vi "CameraVision_Demo_v03.vi"() -> (4 "图像时间戳":u32=16532020 format="%_32g")   [LabVIEW 2015]
uses:
  MVCAMSDK.dll
  <vilib>/Analysis/NI_AALBase.lvlib
  <vilib>/Analysis/NI_AAL_SigProc.lvlib
panel:
  out "泰伯距离数值 3":dbl[](array[numeric])=[15.393849374426454, 15.239052716055017, 15.197063981826837, 15.002070246239633]
  out "Locations 3":dbl[](array[numeric])=[10.438621227921368, 25.832470602347822, 41.07152331840284, 56.268587300229676, 71.27065754646931] caption="上面图像曲线波峰位置"
  out "找到的波谷 2":i32=5
  out "找到的波峰 2":i32=5
  in  "波峰检测器宽度 2":i32=5 min=3
  out "相机每次行进距离  3":dbl=0.1 format="%.2f"
  in  "单次输入步进电机脉冲数  2":i32=20
  out "相机每次行进距离":dbl=0.1 format="%.2f"
  in  "单次输入步进电机脉冲数":i32=20
  out "泰伯距离数值":dbl[](array[numeric])=[15.393849374426454, 15.239052716055017, 15.197063981826837, 15.002070246239633]
  out "Locations":dbl[](array[numeric])=[10.438621227921368, 25.832470602347822, 41.07152331840284, 56.268587300229676, 71.27065754646931] caption="上面图像曲线波峰位置"
  out "找到的波谷":i32=5
  out "找到的波峰":i32=5
  out "信号曲线":cluster{"Locations":dbl[], "Amplitudes":dbl[]}[](graph)=[{"Locations"=array[750 elements], "Amplitudes"=array[749 elements]}, {"Locations"=[104.38621227921368, 258.3247060234782, 410.71523318402836, 562.6858730022967, 712.7065754646931], "Amplitudes"=[11153.698204083417, 10559.387052180104, 10974.865031894917, 10500.852817232146, 11059.763900010517]}, {"Locations"=[26.787398227992274, 182.39455189327623, 333.5517219531509, 488.1851999460032, 636.5270621135614], "Amplitudes"=[3284.809720018355, 2039.4564261182056, 3638.2587716464914, 3082.2730888167225, 4217.856016996603]}]
  in  "波峰检测器宽度":i32=5 min=3
  out "variance 2":dbl caption="方差2" format="%0.2f"
  out "光强图 2":u64[](graph)
  out "variance":dbl caption="方差" format="%0.2f"
  out "相机图像":T1(plugin-control)
  out "光强图":u64[](graph)
  in  "自定义分辨率设置":bool
  in  "ROI分辨率":T2
  in  "预设分辨率设置":bool
  in  "预设分辨率":T3(radio)
  out "帧速":u32
  out "帧间耗时\n单位：（0.1ms）":u32
  in  "相机枚举":T4(ring)
  in  "自动曝光模式":bool=TRUE caption="软触发"
  in  "手动曝光模式":bool caption="软触发"
  in  "曝光时间，单位微秒":dbl=11000.0 format="%#_6f"
  in  "硬触发模式":bool caption="软触发"
  in  "软触发模式":bool caption="软触发"
  in  "连续模式":bool caption="软触发"
  in  "软触发一帧":bool caption="软触发"
  in  "读取自定义数据":bool
  out "从相机中读出的字符串(32字节)":string
  in  "写入自定义数据":bool
  in  "要写入相机的字符串(32字节)":string
  in  "拍照":bool
  in  "相机参数":bool=TRUE
  in  "Stop":bool
  in  "激活预览":bool=TRUE
  out "Image":T1(plugin-control)
  # "相机原生分辨率设置"
  # "写入自定义数据"
  # "触发设置"
  # "曝光设置"
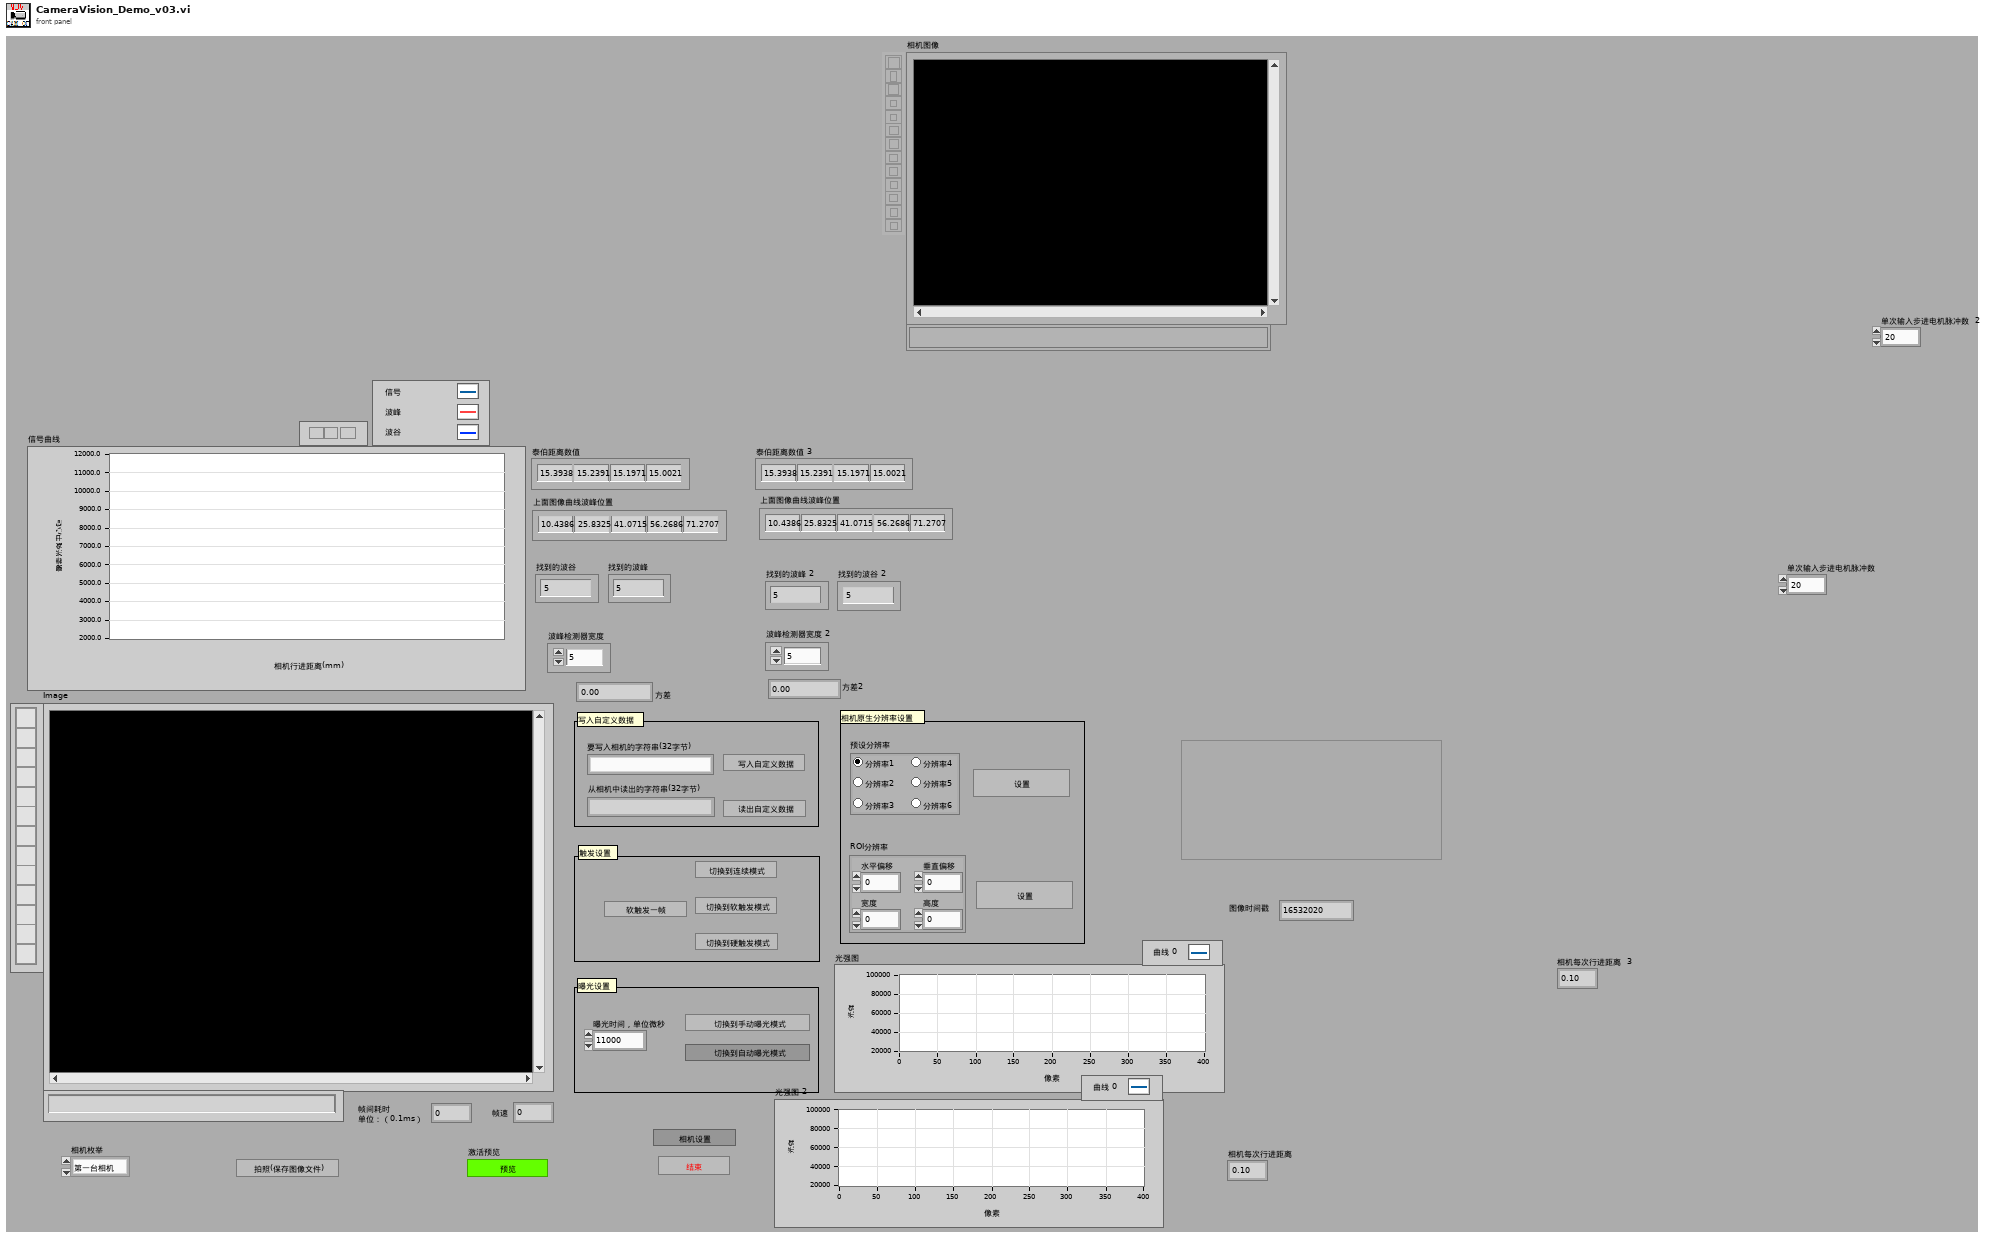
[diagram p1: front panel]
types:
  T1 = typedef "IMAQ Image.ctl" = refnum<image>
  T2 = cluster{"水平偏移":dbl, "垂直偏移":dbl, "宽度":dbl, "高度":dbl}
  T3 = enum32{"分辨率1", "分辨率2", "分辨率3", "分辨率4", "分辨率5", "分辨率6"}
  T4 = enum16{"第一台相机", "第二台相机", "第三台相机", "第四台相机", "第五台相机"}
  T5 = typedef "Image Type" = u32
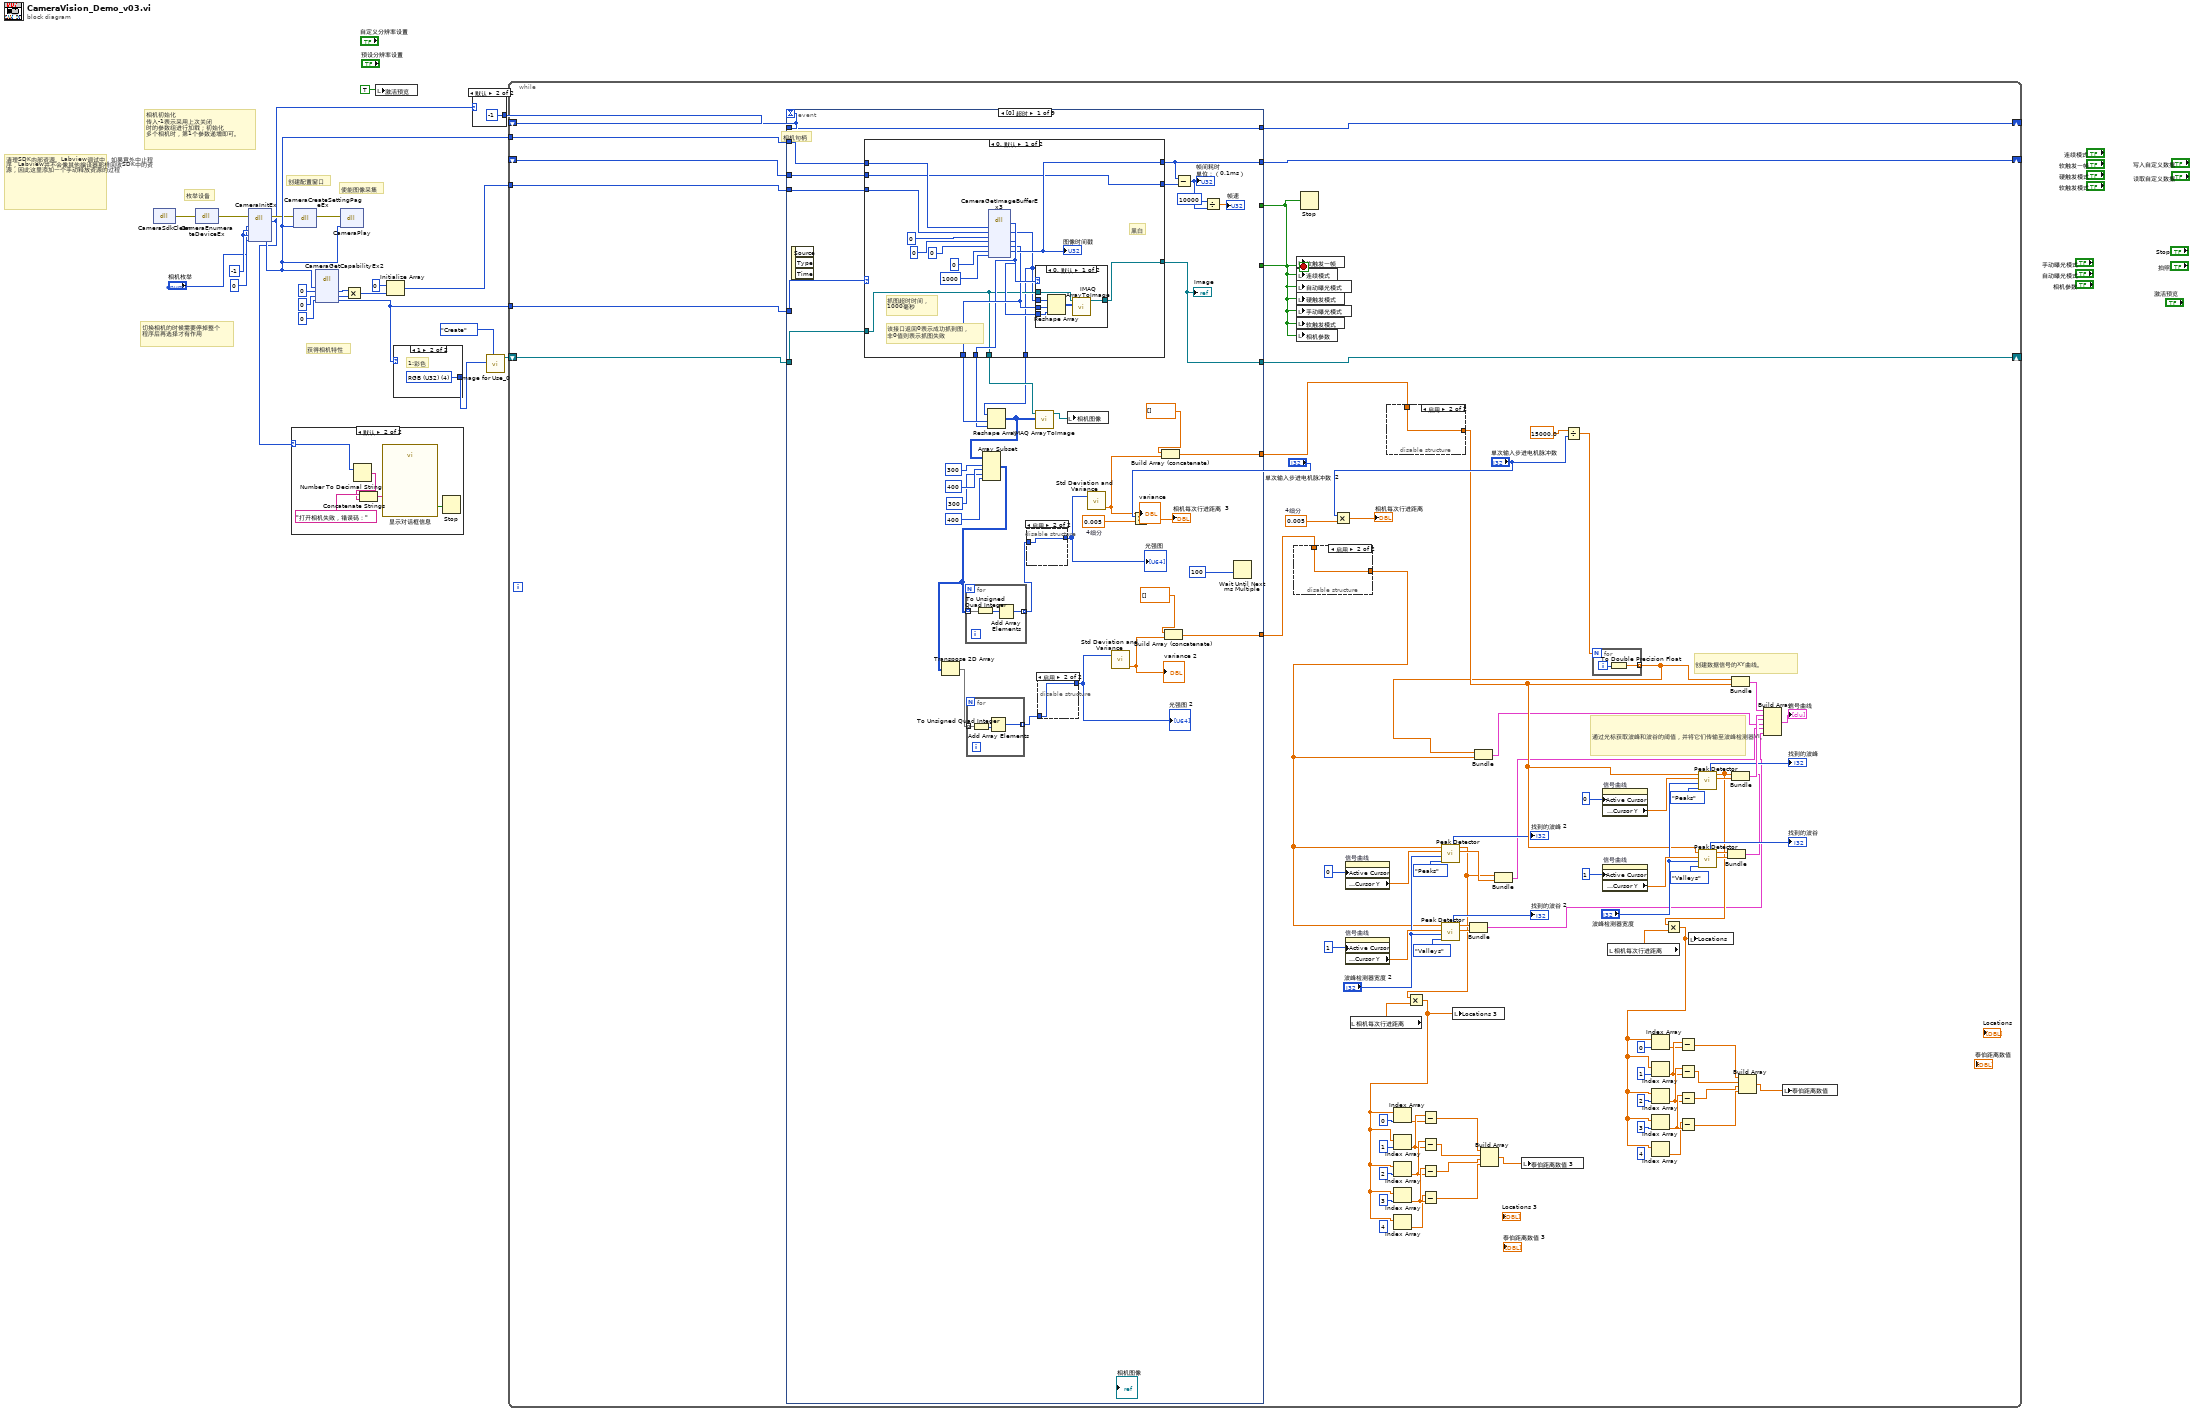
[diagram p0: block diagram]
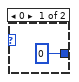
[diagram p2: hidden frame]
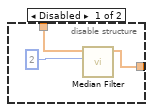
[diagram p4: hidden frame]
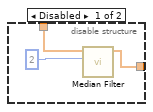
[diagram p5: hidden frame]
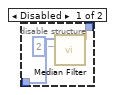
[diagram p6: hidden frame]
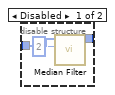
[diagram p7: hidden frame]
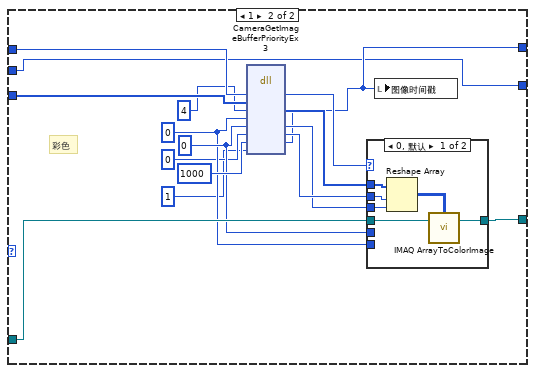
[diagram p9: hidden frame]
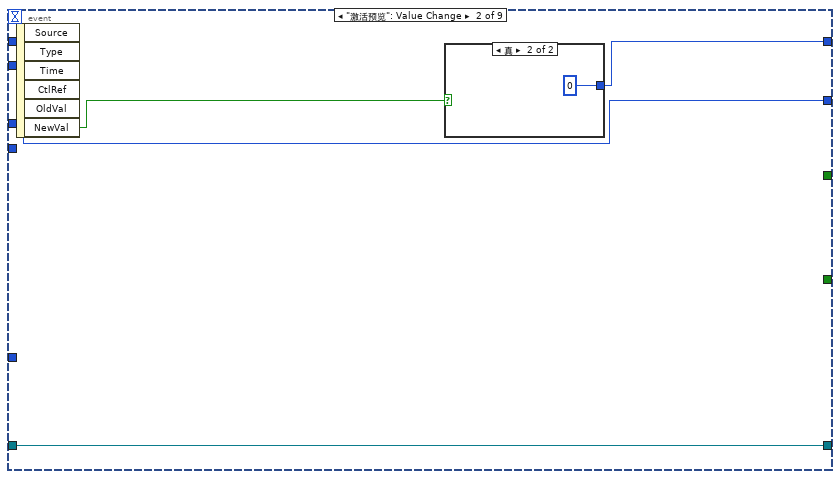
[diagram p11: hidden frame]
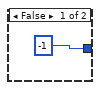
[diagram p12: hidden frame]
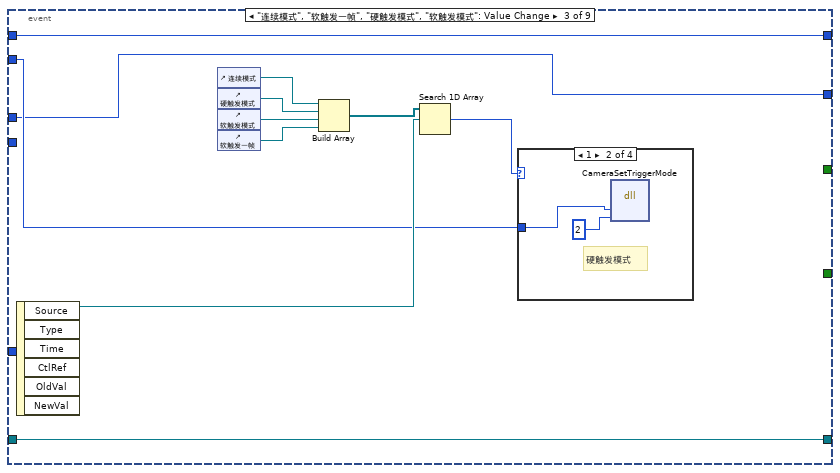
[diagram p13: hidden frame]
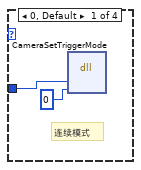
[diagram p14: hidden frame]
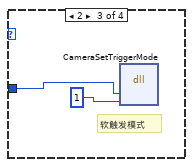
[diagram p15: hidden frame]
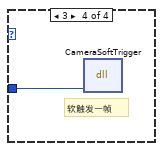
[diagram p16: hidden frame]
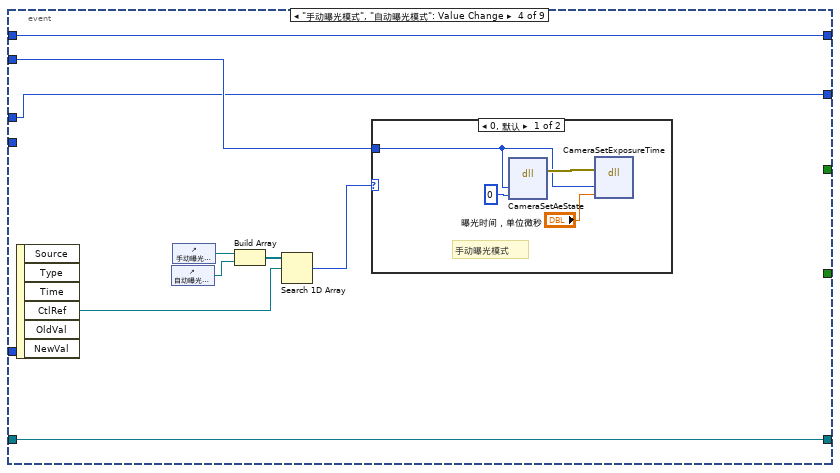
[diagram p17: hidden frame]
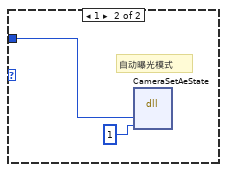
[diagram p18: hidden frame]
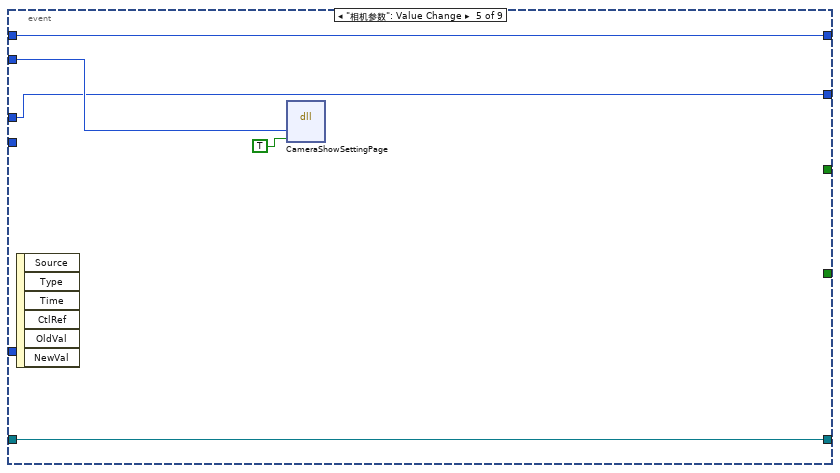
[diagram p19: hidden frame]
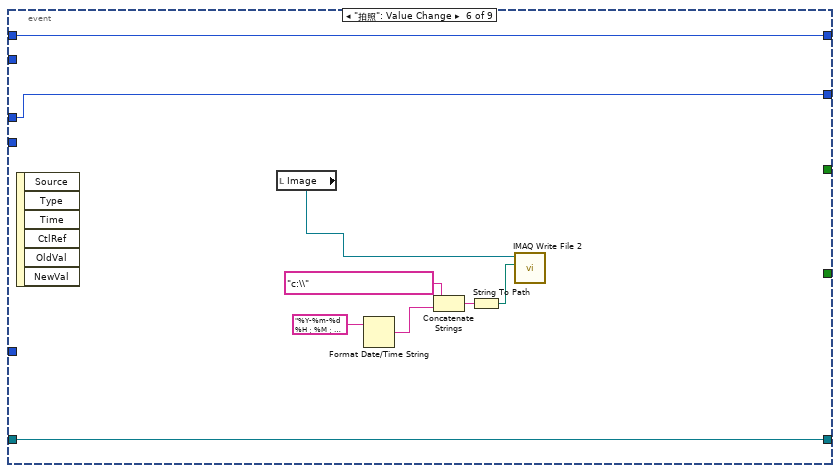
[diagram p20: hidden frame]
diagram:
  w20 = -1
  # "切换相机的时候需要停掉整个\n程序后再选择才有作用"
  # "清理SDK内部资源。Labview调试中，如果意外中止程序，Labview并不会像其他编译器那样回收SDK中的资源，因此这里添加一个手动释放资源的过程"
  # "使能图像采集"
  # "获得相机特性"
  # "创建配置窗口"
  # "相机初始化\n传入-1表示采用上次关闭\n时的参数组进行加载；初始化\n多个相机时，第1个参数递增即可。"
  # "枚举设备"
  n1 = dll-call lib="MVCAMSDK.dll" fn="CameraSdkClean"() -> (error out=w21:errorcluster)  [unwired: 4 in, 1 out]
  n2 = dll-call lib="MVCAMSDK.dll" fn="CameraEnumerateDeviceEx"(error in=w21) -> (error out=w18:errorcluster)  [unwired: 3 in, 1 out]
  n3 = dll-call lib="MVCAMSDK.dll" fn="CameraInitEx"(error in=w18, "相机索引值"="相机枚举", "参数加载方式"=w20, "要加载的参数组索引"=w20, "相机句柄"=0) -> (error out=w7:errorcluster, "返回类型"=w2:i32, "相机句柄"=w9:i32)  [unwired: 5 in, 1 out]
  n4 = case shown="默认" w2 {
    selector: w2 -> [_ w27]
    frame 0 {
    }
    frame Default {
      n5 = Number To Decimal String(number=w27) -> (decimal integer string=w24:string)  [unwired: 1 in]
      n6 = Concatenate Strings("打开相机失败，错误码：" ("字符串"), w24) -> (w26:string)
      n7 = call "显示对话框信息"("Message"=w26) -> ("结束"=w28:bool)  [unwired: 9 in, 1 out]
      n8 = Stop(stop? (T)=w28) -> ()
    }
  }
  n9 = dll-call lib="MVCAMSDK.dll" fn="CameraCreateSettingPageEx"(error in=w7, "相机句柄"=w9) -> (error out=w10:errorcluster)  [unwired: 4 in, 1 out]
  n10 = dll-call lib="MVCAMSDK.dll" fn="CameraGetCapabilityEx2"("相机句柄"=w9, "图像最大宽度"=0, "图像最大高度"=0, "是否是彩色相机(返回0:黑白;1:彩色)"=0) -> ("图像最大宽度"=w12:i32, "图像最大高度"=w11:i32, "是否是彩色相机(返回0:黑白;1:彩色)"=w6:i32)  [unwired: 5 in, 2 out]
  n11 = dll-call lib="MVCAMSDK.dll" fn="CameraPlay"(error in=w10, "相机句柄"=w9) -> ()  [unwired: 4 in, 2 out]
  n12 = Multiply(x=w12, y=w11) -> (x*y=w16:i32)
  n13 = local write "激活预览"(TRUE ("激活预览")) -> ()
  n14 = Initialize Array(0, w16) -> (w8:i32[])
  n15 = case shown="1" w6 {
    tunnel: [_ w29] -> w22
    frame 0, Default {
      # "0:黑白;"
    }
    frame 1 {
      w29 = T5 4 items=["Grayscale (U8)", "Grayscale (I16)", "Grayscale (SGL)", "Complex (CSG)", "RGB (U32)", "HSL (U32)", "RGB (U64)", "Grayscale (U16)"] ("Image Type")
      # "1:彩色"
    }
  }
  n16 = case shown="默认" w2 {
    tunnel: [0 -1] -> w1
    frame 0 {
    }
    frame Default {
    }
  }
  n17 = call "Image for Use_0.vi"("Command"=enum16{"Create", "Use", "Copy in", "Dispose"}."Create", "Image Type"=w22) -> ("Image out"=w5:T1)  [unwired: 8 in, 1 out]
  n18 = while {
    tunnel: w9 -> [w117]
    tunnel: w8 -> [w119]
    tunnel: w6 -> [w120]
    shift-right: [w116] -> _
    shift-left: w1 -> [w115]
    shift-right: [w113] -> _
    shift-left: w5 -> [w118]
    shift-right: [w112] -> _
    shift-left: _ -> [w111]
    stop <- w110 stop-if-true
    (unwired) 4 ("索引")
    w70 = 0.005  # 4细分
    w74 = 0.005  # 4细分
    (unwired) 4 ("索引")
    # "通过光标获取波峰和波谷的阈值，并将它们传输至波峰检测器VI。"
    # "创建数据信号的XY曲线。"
    # "相机句柄"
    n19 = event shown="[0] 超时" {
      selector: _ -> [_ _ _ _ _ _ _ _ _]
      dyn-events: _ -> [_ _ _ _ _ _ _ _ _]
      timeout: w115 -> [_ _ _ _ _ _ _ _ _]
      tunnel: [_ _ _ _ _ _ _ _ TRUE] -> w110
      tunnel: w119 -> [w164 _ _ _ _ _ _ _ _]
      tunnel: w120 -> [w163 _ _ _ _ _ _ _ _]
      tunnel: w117 -> [w165 _ w233 w251 w266 _ w280 w303 w383]
      tunnel: w118 -> [w162 w226 w232 w250 w265 w270 w279 w305 w381]
      tunnel: [w161 w227 w234 w252 w267 w271 w281 w306 w384] -> w116
      tunnel: w115 -> [w161 _ w234 w252 w267 w271 w281 w306 w384]
      tunnel: [_ _ _ _ _ _ _ _ FALSE] -> w114
      tunnel: [w160 w226 w232 w250 w265 w270 w279 w305 w381] -> w113
      tunnel: [w157 w225 w231 w249 w264 w269 w278 w297 w380] -> w112
      tunnel: w111 -> [w159 w225 w231 w249 w264 w269 w278 w297 w380]
      tunnel: [w134 _ _ _ _ _ _ _ _] -> w77
      tunnel: [w131 _ _ _ _ _ _ _ _] -> w67
      event Timeout {
        n20 = event-data() -> ()  [unwired: 1 in, 3 out]
        n21 = case shown="0, 默认" w163 {
          tunnel: w164 -> [w194 w217]
          tunnel: w162 -> [w181 w216]
          tunnel: w165 -> [w186 w215]
          tunnel: [w187 w205] -> w160
          tunnel: [w185 w204] -> w157
          tunnel: w159 -> [w184 w203]
          tunnel: [w184 w203] -> w158
          tunnel: [w183 _] -> w152
          tunnel: [w182 _] -> w151
          tunnel: [w181 _] -> w150
          tunnel: [w180 _] -> w149
          frame 0, Default {
            # "黑白"
            # "该接口返回0表示成功抓到图，\n非0值则表示抓图失败"
            # "抓图超时时间，\n1000毫秒"
            n22 = dll-call lib="MVCAMSDK.dll" fn="CameraGetImageBufferEx3"("相机句柄"=w186, "图像数据缓冲区"=w194, "图像输出格式(0:8位灰度;1:24位彩色;2:32位彩色，3：BGR24彩色 4：BGRA32位彩色)"=0, "图像宽度"=0, "图像高度"=0, "时间戳(单位为100微秒)"=0, "抓图超时时间(毫秒)"=1000) -> ("返回类型"=w189:i32, "图像数据缓冲区"=w180:u8[], "图像宽度"=w182:i32, "图像高度"=w183:i32, "时间戳(单位为100微秒)"=w185:u32)  [unwired: 6 in, 2 out]
            "图像时间戳" <- w185
            n23 = case shown="0, 默认" w189 {
              tunnel: w180 -> [w200 _]
              tunnel: w181 -> [w197 w201]
              tunnel: w183 -> [w199 _]
              tunnel: w182 -> [w198 _]
              tunnel: [w195 w201] -> w187
              frame 0, Default {
                n24 = Reshape Array(w200, w199, w198) -> (w196:u8[][])
                n25 = call "IMAQ ArrayToImage"("Image Pixels (U8)"=w196, "Image"=w197) -> ("Image Out"=w195:T1)  [unwired: 8 in, 1 out]
              }
              frame -12 {
              }
            }
          }
          frame 1 {
            w207 = 0
            w208 = 0
            # "彩色"
            n26 = dll-call lib="MVCAMSDK.dll" fn="CameraGetImageBufferPriorityEx3"("相机句柄"=w215, "图像数据缓冲区"=w217, "图像输出格式(0:8位灰度;1:24位彩色;2:32位彩色)"=4, "图像宽度"=w207, "图像高度"=w208, "时间戳（单位为100微秒）"=0, "抓图超时时间(毫秒)"=1000, "取图优先级(0: 取最旧   1:取最新)"=1) -> ("返回类型"=w209:i32, "图像数据缓冲区"=w212:u32[], "图像宽度"=w210:i32, "图像高度"=w211:i32, "时间戳（单位为100微秒）"=w204:u32)  [unwired: 7 in, 2 out]
            n27 = case shown="0, 默认" w209 {
              tunnel: w212 -> [w222 _]
              tunnel: w216 -> [w221 w224]
              tunnel: w211 -> [w220 _]
              tunnel: w210 -> [w219 _]
              tunnel: w208 -> [_ _]
              tunnel: w207 -> [_ _]
              tunnel: [w218 w224] -> w205
              frame 0, Default {
                n28 = Reshape Array(w222, w220, w219) -> (w223:u32[][])
                n29 = call "IMAQ ArrayToColorImage"("Image Pixels (U32)"=w223, "Image"=w221) -> ("Image Out"=w218:T1)  [unwired: 3 in, 1 out]
              }
              frame -12 {
              }
            }
            n30 = local write "图像时间戳"(w204) -> ()
          }
        }
        "Image" <- w160
        n31 = Reshape Array(w149, w152, w151) -> (w138:u8[][])
        n32 = Array Subset(array=w138, index (row)=300 ("索引"), length (row)=400 ("长度"), index (col)=300 ("长度"), length (col)=400 ("索引")) -> (w137:u8[][])
        n33 = Transpose 2D Array(2D array=w137) -> (transposed array=w145:u8[][])
        n34 = for {
          tunnel: w137 -> [w174] mode=indexing
          tunnel: [w175] -> w147 mode=indexing
          n35 = To Unsigned Quad Integer(1:w174) -> (0:w173:u64[])
          n36 = Add Array Elements(numeric array=w173) -> (sum=w175:u64)
        }
        n37 = for {
          tunnel: w145 -> [w167] mode=indexing
          tunnel: [w168] -> w146 mode=indexing
          n38 = To Unsigned Quad Integer(1:w167) -> (0:w166:u64[])
          n39 = Add Array Elements(numeric array=w166) -> (sum=w168:u64)
        }
        n40 = disable-structure shown="启用" {
          disable-tunnel: w147 -> [w178 w179]
          disable-tunnel: [w176 w179] -> w144
          frame Disabled {
            n41 = call <vilib>:"Median Filter.vi"("left rank"=2, "X"=w178) -> ("Filtered X"=w176:dbl[])  [unwired: 8 in, 1 out]
          }
          frame Enabled {
          }
        }
        "光强图" <- w144
        n42 = call "IMAQ ArrayToImage"("Image Pixels (U8)"=w138, "Image"=w150) -> ("Image Out"=w153:T1)  [unwired: 8 in, 1 out]
        n43 = disable-structure shown="启用" {
          disable-tunnel: w146 -> [w171 w172]
          disable-tunnel: [w169 w172] -> w143
          frame Disabled {
            n44 = call <vilib>:"Median Filter.vi"("left rank"=2, "X"=w171) -> ("Filtered X"=w169:dbl[])  [unwired: 8 in, 1 out]
          }
          frame Enabled {
          }
        }
        "光强图 2" <- w143
        n45 = local write "相机图像"(w153) -> ()
        n46 = call <vilib>:"Std Deviation and Variance.vi"("X"=w144) -> ("variance"=w136:dbl)  [unwired: 1 in, 2 out]
        "variance" <- w136
        n47 = call <vilib>:"Std Deviation and Variance.vi"("X"=w143) -> ("variance"=w132:dbl)  [unwired: 1 in, 2 out]
        "variance 2" <- w132
        n48 = Build Array (concatenate)(dbl[] [], w136) -> (w134:dbl[])
        n49 = Build Array (concatenate)(dbl[] [], w132) -> (w131:dbl[])
        n50 = Subtract(x=w157, y=w158) -> (x-y=w156:u32)
        "帧间耗时\n单位：（0.1ms）" <- w156
        n51 = Divide(x=u32 10000 ("帧间耗时"), y=w156) -> (x/y=→"帧速":dbl)
        n52 = Wait Until Next ms Multiple(millisecond multiple=u32 100 ("毫秒倍数")) -> ()  [unwired: 1 out]
      }
      event "激活预览": Value Change {
        n53 = event-data() -> ("NewVal"=w228:bool)  [unwired: 1 in, 5 out]
        n54 = case shown="真" w228 {
          tunnel: [-1 0] -> w227
          frame False {
          }
          frame True {
          }
        }
      }
      event "连续模式", "软触发一帧", "硬触发模式", "软触发模式": Value Change {
        n55 = event-data() -> ("CtlRef"=w236:refnum<vi>)  [unwired: 1 in, 5 out]
        n56 = control-ref of="连续模式"() -> (w238:refnum<vi>)
        n57 = control-ref of="硬触发模式"() -> (w239:refnum<vi>)
        n58 = control-ref of="软触发模式"() -> (w240:refnum<vi>)
        n59 = control-ref of="软触发一帧"() -> (w241:refnum<vi>)
        n60 = Build Array ("创建数组")(w238, w239, w240, w241) -> (w237:refnum<vi>[])
        n61 = Search 1D Array(1D array=w237, element=w236) -> (index of element=w235:i32)  [unwired: 1 in]
        n62 = case shown="1" w235 {
          tunnel: w233 -> [w242 w244 w246 w248]
          frame 0, Default {
            # "连续模式"
            n63 = dll-call lib="MVCAMSDK.dll" fn="CameraSetTriggerMode"("相机句柄"=w242, "模式"=0) -> ()  [unwired: 6 in, 2 out]
          }
          frame 1 {
            # "硬触发模式"
            n64 = dll-call lib="MVCAMSDK.dll" fn="CameraSetTriggerMode"("相机句柄"=w244, "模式"=2) -> ()  [unwired: 6 in, 2 out]
          }
          frame 2 {
            # "软触发模式"
            n65 = dll-call lib="MVCAMSDK.dll" fn="CameraSetTriggerMode"("相机句柄"=w246, "模式"=1) -> ()  [unwired: 6 in, 2 out]
          }
          frame 3 {
            # "软触发一帧"
            n66 = dll-call lib="MVCAMSDK.dll" fn="CameraSoftTrigger"("相机句柄"=w248) -> ()  [unwired: 5 in, 2 out]
          }
        }
      }
      event "手动曝光模式", "自动曝光模式": Value Change {
        n67 = event-data() -> ("CtlRef"=w255:refnum<vi>)  [unwired: 1 in, 5 out]
        n68 = control-ref of="自动曝光模式"() -> (w253:refnum<vi>)
        n69 = control-ref of="手动曝光模式"() -> (w256:refnum<vi>)
        n70 = Build Array ("创建数组")(w256, w253) -> (w257:refnum<vi>[])
        n71 = Search 1D Array(1D array=w257, element=w255) -> (index of element=w254:i32)  [unwired: 1 in]
        n72 = case shown="0, 默认" w254 {
          tunnel: w251 -> [w258 w262]
          frame 0, Default {
            # "手动曝光模式"
            n73 = dll-call lib="MVCAMSDK.dll" fn="CameraSetAeState"("相机句柄"=w258, "曝光模式(0手动，1自动)"=0) -> (error out=w261:errorcluster)  [unwired: 6 in, 1 out]
            n74 = dll-call lib="MVCAMSDK.dll" fn="CameraSetExposureTime"(error in=w261, "相机句柄"=w258, "曝光时间，单位微秒"="曝光时间，单位微秒") -> ()  [unwired: 5 in, 2 out]
          }
          frame 1 {
            # "自动曝光模式"
            n75 = dll-call lib="MVCAMSDK.dll" fn="CameraSetAeState"("相机句柄"=w262, "曝光模式(0手动，1自动)"=1) -> ()  [unwired: 6 in, 2 out]
          }
        }
      }
      event "相机参数": Value Change {
        n76 = event-data() -> ()  [unwired: 1 in, 6 out]
        n77 = dll-call lib="MVCAMSDK.dll" fn="CameraShowSettingPage"("相机句柄"=w266, "状态"=TRUE) -> ()  [unwired: 6 in, 2 out]
      }
      event "拍照": Value Change {
        n78 = event-data() -> ()  [unwired: 1 in, 6 out]
        n79 = local read "Image"() -> (w272:T1)
        n80 = Format Date/Time String(time format string (%c)="%Y-%m-%d %H：%M：%S.bmp ") -> (date/time string=w276:string)  [unwired: 2 in]
        n81 = Concatenate Strings("c:\\", w276) -> (w273:string)
        n82 = String To Path(string=w273) -> (path=w275:path)
        n83 = call-poly "IMAQ Write File 2"("File Path"=w275, "Image"=w272) -> ()  [unwired: 8 in, 2 out]
      }
      event "写入自定义数据", "读取自定义数据": Value Change {
        n84 = event-data() -> ("CtlRef"=w283:refnum<vi>)  [unwired: 1 in, 5 out]
        n85 = control-ref of="读取自定义数据"() -> (w285:refnum<vi>)
        n86 = control-ref of="写入自定义数据"() -> (w284:refnum<vi>)
        n87 = Build Array ("创建数组")(w285, w284) -> (w286:refnum<vi>[])
        n88 = Search 1D Array(1D array=w286, element=w283) -> (index of element=w282:i32)  [unwired: 1 in]
        n89 = case shown="0, 默认" w282 {
          tunnel: w280 -> [w287 w294]
          frame 0, Default {
            n90 = Initialize Array(0, 32) -> (w291:i32[])
            n91 = dll-call lib="MVCAMSDK.dll" fn="CameraReadSN"("相机句柄"=w287, "序列号"=w291, "序列号级别，[0,1,2],0级为只读，1,2级可写"=1) -> ("序列号"=w289:u8[])  [unwired: 6 in, 2 out]
            n92 = Byte Array To String(unsigned byte array=w289) -> (string=→"从相机中读出的字符串(32字节)":string)
          }
          frame 1 {
            n93 = dll-call lib="MVCAMSDK.dll" fn="CameraWriteSN"("相机句柄"=w294, "序列号(固定为32个字节)"="要写入相机的字符串(32字节)", "序列号级别，[0,1,2]对应3级序列号，其中0级为只读，1,2级可写"=1) -> ()  [unwired: 7 in, 2 out]
          }
        }
      }
      event "预设分辨率设置", "自定义分辨率设置": Value Change {
        n94 = event-data() -> ("CtlRef"=w299:refnum<vi>)  [unwired: 1 in, 5 out]
        n95 = control-ref of="预设分辨率设置"() -> (w301:refnum<vi>)
        n96 = control-ref of="自定义分辨率设置"() -> (w300:refnum<vi>)
        n97 = Build Array ("创建数组")(w301, w300) -> (w302:refnum<vi>[])
        n98 = Search 1D Array(1D array=w302, element=w299) -> (index of element=w298:i32)  [unwired: 1 in]
        n99 = case shown="1" w298 {
          tunnel: "预设分辨率" -> [w308 _]
          tunnel: w303 -> [w307 w369]
          frame 0, Default {
            n100 = case shown="\"分辨率2\"" w308 {
              tunnel: w307 -> [w309 w328 w329 w339 w349 w359]
              frame "分辨率1", Default {
                n101 = dll-call lib="MVCAMSDK.dll" fn="CameraSetImageResolutionEx"("相机句柄"=w309, "预设分辨率索引"=0, "Mode"=0, "ModeSize"=u32 0, "x"=0, "y"=u32 0 ("ModeSize"), "width"=0, "height"=0, "ZoomWidth"=0, "ZoomHeight"=0) -> ()  [unwired: 14 in, 2 out]
              }
              frame "分辨率2" {
                n102 = dll-call lib="MVCAMSDK.dll" fn="CameraSetImageResolutionEx"("相机句柄"=w328, "预设分辨率索引"=1, "Mode"=0, "ModeSize"=u32 0, "x"=0, "y"=u32 0 ("ModeSize"), "width"=0, "height"=0, "ZoomWidth"=0, "ZoomHeight"=0) -> ()  [unwired: 14 in, 2 out]
              }
              frame "分辨率3" {
                n103 = dll-call lib="MVCAMSDK.dll" fn="CameraSetImageResolutionEx"("相机句柄"=w329, "预设分辨率索引"=2, "Mode"=0, "ModeSize"=u32 0, "x"=0, "y"=u32 0 ("ModeSize"), "width"=0, "height"=0, "ZoomWidth"=0, "ZoomHeight"=0) -> ()  [unwired: 14 in, 2 out]
              }
              frame "分辨率4" {
                n104 = dll-call lib="MVCAMSDK.dll" fn="CameraSetImageResolutionEx"("相机句柄"=w339, "预设分辨率索引"=3, "Mode"=0, "ModeSize"=u32 0, "x"=0, "y"=u32 0 ("ModeSize"), "width"=0, "height"=0, "ZoomWidth"=0, "ZoomHeight"=0) -> ()  [unwired: 14 in, 2 out]
              }
              frame "分辨率5" {
                n105 = dll-call lib="MVCAMSDK.dll" fn="CameraSetImageResolutionEx"("相机句柄"=w349, "预设分辨率索引"=4, "Mode"=0, "ModeSize"=u32 0, "x"=0, "y"=u32 0 ("ModeSize"), "width"=0, "height"=0, "ZoomWidth"=0, "ZoomHeight"=0) -> ()  [unwired: 14 in, 2 out]
              }
              frame "分辨率6" {
                n106 = dll-call lib="MVCAMSDK.dll" fn="CameraSetImageResolutionEx"("相机句柄"=w359, "预设分辨率索引"=5, "Mode"=0, "ModeSize"=u32 0, "x"=0, "y"=u32 0 ("ModeSize"), "width"=0, "height"=0, "ZoomWidth"=0, "ZoomHeight"=0) -> ()  [unwired: 14 in, 2 out]
              }
            }
          }
          frame 1 {
            n107 = Unbundle("ROI分辨率") -> ("水平偏移"=w371:dbl, "垂直偏移"=w372:dbl, "宽度"=w373:dbl, "高度"=w374:dbl)
            n108 = dll-call lib="MVCAMSDK.dll" fn="CameraSetImageResolutionEx"("相机句柄"=w369, "预设分辨率索引"=255, "Mode"=0, "ModeSize"=u32 0, "x"=w371, "y"=w372, "width"=w373, "height"=w374, "ZoomWidth"=0, "ZoomHeight"=u32 0 ("ModeSize")) -> ()  [unwired: 14 in, 2 out]
          }
        }
      }
      event "Stop": Value Change {
        # "反初始化相机"
        n109 = event-data() -> ()  [unwired: 1 in, 6 out]
        n110 = dll-call lib="MVCAMSDK.dll" fn="CameraUnInit"("相机句柄"=w383) -> ()  [unwired: 5 in, 2 out]
      }
    }
    n111 = Multiply(x="单次输入步进电机脉冲数  2", y=w70) -> (x*y=→"相机每次行进距离  3":dbl)
    n112 = disable-structure shown="启用" {
      disable-tunnel: w67 -> [w122 w124]
      disable-tunnel: [w121 w124] -> w36
      frame Disabled {
        n113 = call <vilib>:"Median Filter.vi"("left rank"=2, "X"=w122) -> ("Filtered X"=w121:dbl[])  [unwired: 8 in, 1 out]
      }
      frame Enabled {
      }
    }
    n114 = local write "软触发一帧"(w114) -> ()
    n115 = local write "连续模式"(w114) -> ()
    n116 = local write "自动曝光模式"(w114) -> ()
    n117 = local write "硬触发模式"(w114) -> ()
    n118 = local write "手动曝光模式"(w114) -> ()
    n119 = local write "软触发模式"(w114) -> ()
    n120 = local write "相机参数"(w114) -> ()
    n121 = Stop(stop? (T)=w110) -> ()
    n122 = Multiply(x="单次输入步进电机脉冲数", y=w74) -> (x*y=→"相机每次行进距离":dbl)
    n123 = property on="信号曲线" class="XYGraph (严格)"("Active Cursor"=u32 0) -> ("Cursor.Cursor Position:Cursor Y"=w60:dbl)  [unwired: 2 in, 2 out]
    n124 = property on="信号曲线" class="XYGraph (严格)"("Active Cursor"=u32 1) -> ("Cursor.Cursor Position:Cursor Y"=w59:dbl)  [unwired: 2 in, 2 out]
    n125 = local read "相机每次行进距离"() -> (w53:dbl)
    n126 = disable-structure shown="启用" {
      disable-tunnel: w77 -> [w128 w130]
      disable-tunnel: [w127 w130] -> w71
      frame Disabled {
        n127 = call <vilib>:"Median Filter.vi"("left rank"=2, "X"=w128) -> ("Filtered X"=w127:dbl[])  [unwired: 8 in, 1 out]
      }
      frame Enabled {
      }
    }
    n128 = call <vilib>:"Peak Detector.vi"("peaks/valleys"=enum32{"Peaks", "Valleys"}."Peaks", "width"="波峰检测器宽度 2", "threshold"=w60, "X"=w36) -> ("Amplitudes"=w64:dbl[], "Locations"=w37:dbl[], "# found"=→"找到的波峰 2":i32)  [unwired: 3 in, 2 out]
    n129 = Multiply(x=w37, y=w53) -> (x*y=w40:dbl[])
    n130 = Index Array(array=w40, index=0 ("索引")) -> (element=w45:dbl)
    n131 = Index Array(array=w40, index=1 ("索引")) -> (element=w46:dbl)
    n132 = Index Array(array=w40, index=2 ("索引")) -> (element=w47:dbl)
    n133 = Index Array(array=w40, index=3 ("索引")) -> (element=w48:dbl)
    n134 = Index Array(array=w40) -> (element=w38:dbl)  [unwired: 1 in]
    n135 = Subtract(x=w46, y=w45) -> (x-y=w49:dbl)
    n136 = Subtract(x=w47, y=w46) -> (x-y=w50:dbl)
    n137 = Subtract(x=w48, y=w47) -> (x-y=w51:dbl)
    n138 = Subtract(x=w38, y=w48) -> (x-y=w52:dbl)
    n139 = call <vilib>:"Peak Detector.vi"("peaks/valleys"=enum32{"Peaks", "Valleys"}."Valleys", "width"="波峰检测器宽度 2", "threshold"=w59, "X"=w36) -> ("Amplitudes"=w62:dbl[], "Locations"=w63:dbl[], "# found"=→"找到的波谷 2":i32)  [unwired: 3 in, 2 out]
    n140 = local write "Locations 3"(w40) -> ()
    n141 = Bundle("Locations"=w63, "Amplitudes"=w62) -> (w33:cluster{"Locations":dbl[], "Amplitudes":dbl[]})  [unwired: 1 in]
    n142 = Build Array(w49, w50, w51, w52) -> (w39:dbl[])
    n143 = Bundle("Locations"=w37, "Amplitudes"=w64) -> (w34:cluster{"Locations":dbl[], "Amplitudes":dbl[]})  [unwired: 1 in]
    n144 = local write "泰伯距离数值 3"(w39) -> ()
    n145 = Divide(x=15000.0 ("y"), y="单次输入步进电机脉冲数") -> (x/y=w76:dbl)
    n146 = for {
      N: w76 -> [_]
      tunnel: [w125] -> w35 mode=indexing
      i -> [w126]
      n147 = To Double Precision Float(number=w126) -> (double precision float=w125:dbl)
    }
    n148 = Bundle(w35, w36) -> (w32:cluster{dbl[], dbl[]})  [unwired: 1 in]
    n149 = property on="信号曲线" class="XYGraph (严格)"("Active Cursor"=u32 0) -> ("Cursor.Cursor Position:Cursor Y"=w101:dbl)  [unwired: 2 in, 2 out]
    n150 = property on="信号曲线" class="XYGraph (严格)"("Active Cursor"=u32 1) -> ("Cursor.Cursor Position:Cursor Y"=w100:dbl)  [unwired: 2 in, 2 out]
    n151 = local read "相机每次行进距离"() -> (w93:dbl)
    n152 = call <vilib>:"Peak Detector.vi"("peaks/valleys"=enum32{"Peaks", "Valleys"}."Peaks", "width"="波峰检测器宽度", "threshold"=w101, "X"=w71) -> ("Amplitudes"=w107:dbl[], "Locations"=w75:dbl[], "# found"=→"找到的波峰":i32)  [unwired: 3 in, 2 out]
    n153 = Multiply(x=w75, y=w93) -> (x*y=w80:dbl[])
    n154 = Index Array(array=w80, index=0 ("索引")) -> (element=w85:dbl)
    n155 = Index Array(array=w80, index=1 ("索引")) -> (element=w86:dbl)
    n156 = Index Array(array=w80, index=2 ("索引")) -> (element=w87:dbl)
    n157 = Index Array(array=w80, index=3 ("索引")) -> (element=w88:dbl)
    n158 = Index Array(array=w80) -> (element=w78:dbl)  [unwired: 1 in]
    n159 = Subtract(x=w86, y=w85) -> (x-y=w89:dbl)
    n160 = Subtract(x=w87, y=w86) -> (x-y=w90:dbl)
    n161 = Subtract(x=w88, y=w87) -> (x-y=w91:dbl)
    n162 = Subtract(x=w78, y=w88) -> (x-y=w92:dbl)
    n163 = local write "Locations"(w80) -> ()
    n164 = call <vilib>:"Peak Detector.vi"("peaks/valleys"=enum32{"Peaks", "Valleys"}."Valleys", "width"="波峰检测器宽度", "threshold"=w100, "X"=w71) -> ("Amplitudes"=w104:dbl[], "Locations"=w105:dbl[], "# found"=→"找到的波谷":i32)  [unwired: 3 in, 2 out]
    n165 = Bundle("Locations"=w105, "Amplitudes"=w104) -> (w66:cluster{"Locations":dbl[], "Amplitudes":dbl[]})  [unwired: 1 in]
    n166 = Bundle(w35, w71) -> (w109:cluster{dbl[], dbl[]})  [unwired: 1 in]
    n167 = Bundle("Locations"=w75, "Amplitudes"=w107) -> (w106:cluster{"Locations":dbl[], "Amplitudes":dbl[]})  [unwired: 1 in]
    n168 = Build Array(w89, w90, w91, w92) -> (w79:dbl[])
    n169 = Build Array(w109, w106, w66, w32, w34, w33) -> (→"信号曲线":cluster{"Locations":dbl[], "Amplitudes":dbl[]}[])
    n170 = local write "泰伯距离数值"(w79) -> ()
  }
